vi "ConvertSlotToString.vi"(11 "Slot":T1) -> (3 "Slot":string)   [LabVIEW 2012, in "Keithley-7001.lvlib"]
uses:
  Keithley-7001.lvlib
  Public/Controls/Slot.ctl
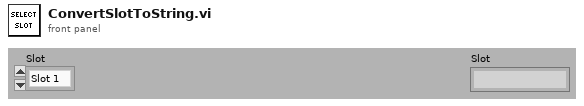
[diagram p1: front panel]
types:
  T1 = typedef "Keithley-7001.lvlib/Slot.ctl" = enum16{"Slot 1", "Slot 2"}
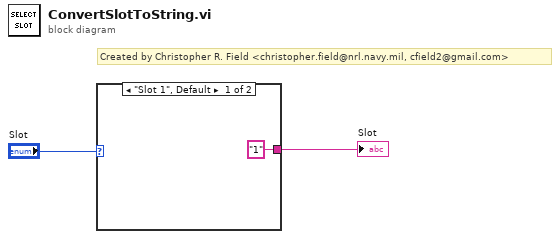
[diagram p0: block diagram]
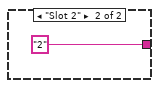
[diagram p2: hidden frame]
diagram:
  # "Created by Christopher R. Field <christopher.field@nrl.navy.mil, cfield2@gmail.com>"
  n1 = case shown="\"Slot 1\", Default" "Slot" {
    tunnel: ["1" "2"] -> w1
    frame "Slot 1", Default {
    }
    frame "Slot 2" {
    }
  }
  "Slot" <- w1
